vi "3shot.vi"() -> (3 "Outputs":T2)   [LabVIEW 2012]
uses:
  util/Outputs.ctl
  mecanum/mecanum_output.ctl
  shooter/shooter_outputs.ctl
  climber/climber_outputs.ctl
  shooter/shooter_cmds.ctl
panel:
  in  "Shooter":T1
  in  "Outputs 2":T2
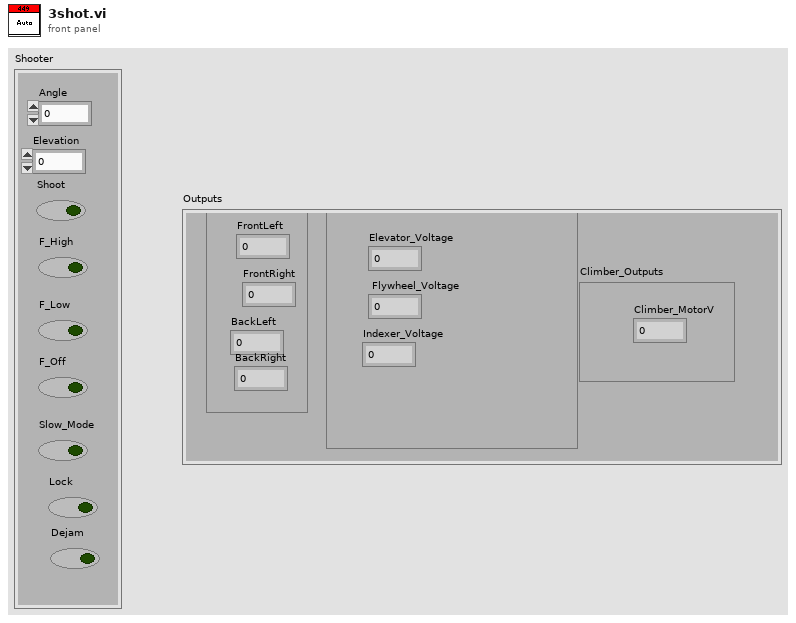
[diagram p1: front panel]
types:
  T1 = typedef "shooter_cmds.ctl" = cluster{"Elevation":dbl, "Shoot":bool, "F_High":bool, "F_Low":bool, "F_Off":bool, "Slow_Mode":bool, "Lock":bool, "Dejam":bool, "Angle":dbl}
  T2 = typedef "Outputs.ctl" = cluster{"Mecanum":T3, "Shooter_Outputs":T4, "Climber_Outputs":T5}
  T3 = typedef "mecanum_output.ctl" = cluster{"FrontLeft":dbl, "FrontRight":dbl, "BackLeft":dbl, "BackRight":dbl}
  T4 = typedef "shooter_outputs.ctl" = cluster{"Elevator_Voltage":dbl, " Flywheel_Voltage":dbl, "Indexer_Voltage":dbl}
  T5 = typedef "climber_outputs.ctl" = cluster{"Climber_MotorV":dbl}
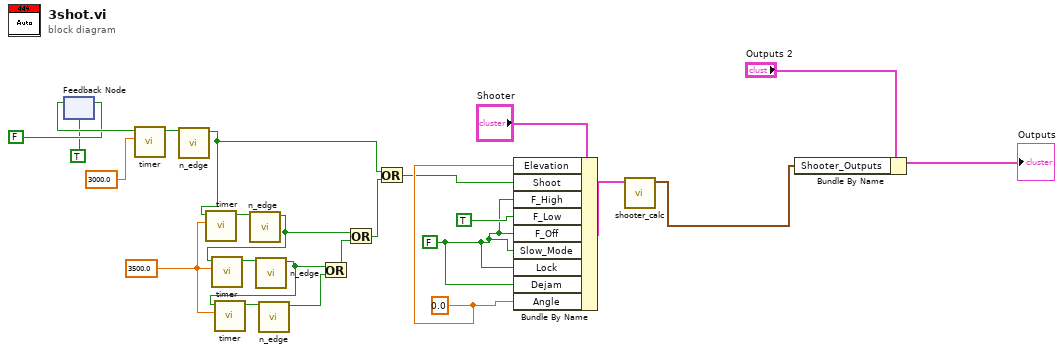
[diagram p0: block diagram]
diagram:
  w1 = 3500.0 ("Time")
  w17 = 0.0 ("Angle")
  w18 = FALSE ("F_Off")
  n1 = feedback-in #1(FALSE) -> ()
  n2 = feedback #1(TRUE) -> (w16:bool)
  n3 = call "timer.vi"("Time"=3000.0, "In"=w16) -> ("Out"=w13:bool)  [unwired: 9 in]
  n4 = call "n_edge.vi"("in"=w13) -> ("out"=w9:bool)  [unwired: 10 in]
  n5 = call "timer.vi"("Time"=w1, "In"=w9) -> ("Out"=w12:bool)  [unwired: 9 in]
  n6 = call "n_edge.vi"("in"=w12) -> ("out"=w8:bool)  [unwired: 10 in]
  n7 = call "timer.vi"("Time"=w1, "In"=w8) -> ("Out"=w11:bool)  [unwired: 9 in]
  n8 = call "n_edge.vi"("in"=w11) -> ("out"=w4:bool)  [unwired: 10 in]
  n9 = call "timer.vi"("Time"=w1, "In"=w4) -> ("Out"=w5:bool)  [unwired: 9 in]
  n10 = call "n_edge.vi"("in"=w5) -> ("out"=w3:bool)  [unwired: 10 in]
  n11 = Or(x=w4, y=w3) -> (x .or. y?=w6:bool)
  n12 = Or(x=w8, y=w6) -> (x .or. y?=w7:bool)
  n13 = Or(x=w9, y=w7) -> (x .or. y?=w10:bool)
  n14 = Bundle By Name(cluster="Shooter", "Elevation"=w17, "Shoot"=w10, "F_High"=w18, "F_Low"=TRUE, "F_Off"=w18, "Slow_Mode"=w18, "Lock"=w18, "Dejam"=w18, "Angle"=w17) -> (w20:T1)
  n15 = call "shooter_calc.vi"("Shooter"=w20) -> ("Shooter_Outputs"=w22:T4)  [unwired: 10 in]
  n16 = Bundle By Name(cluster="Outputs 2", "Shooter_Outputs"=w22) -> (→"Outputs":T2)
